vi "Preview.vi"(8 "error in (no error)":errorcluster, 10 "Project":refnum<vi>, 11 "IB_Tree_Item_Proj_Container in":refnum<class "IB_Tree_Item_Proj_Container.lvclass">) -> (0 "error out":errorcluster, 2 "first preview?":bool, 3 "IB_Tree_Item_Proj_Container out":refnum<class "IB_Tree_Item_Proj_Container.lvclass">)   [LabVIEW 2020, in "IB_Tree_Item_Proj_Container.lvclass"]
uses:
  <vilib>/AppBuilder/IB_Classes/Tree_Item_Proj_Container/IB_Tree_Item_Proj_Container.lvclass
  <vilib>/AppBuilder/IB_Classes/Tree_Item_Proj_Container/IB_Tree_Item_Proj_Container.lvclass/IB_Tree_Item_Proj_Container.ctl
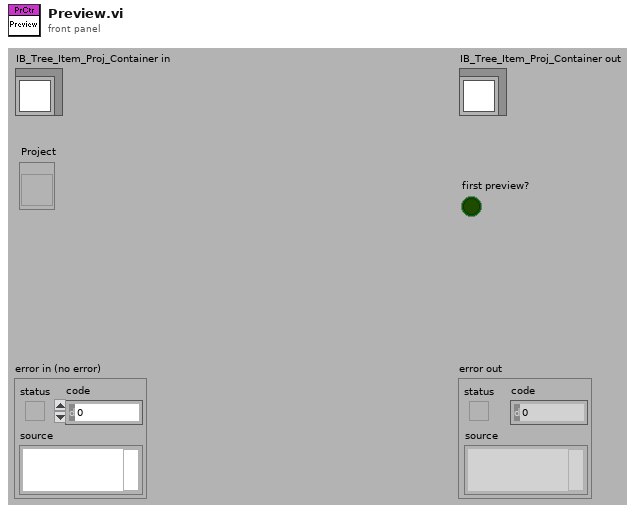
[diagram p1: front panel]
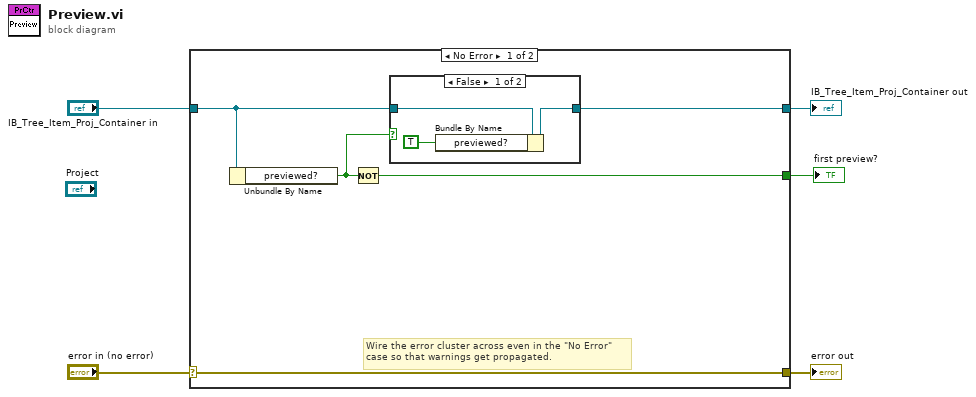
[diagram p0: block diagram]
diagram:
  n1 = case shown="No Error" "error in (no error)" {
    selector: "error in (no error)" -> [w10 w16]
    tunnel: [w10 w16] -> w4
    tunnel: [w8 w15] -> w2
    tunnel: "IB_Tree_Item_Proj_Container in" -> [w9 w15]
    tunnel: [w7 _] -> w1
    frame No Error {
      # "Wire the error cluster across even in the \"No Error\"\ncase so that warnings get propagated."
      n2 = Unbundle By Name(w9) -> ("previewed?"=w6:bool)
      n3 = Not(x=w6) -> (.not. x?=w7:bool)
      n4 = case shown="False" w6 {
        tunnel: w9 -> [w13 w14]
        tunnel: [w12 w14] -> w8
        frame False {
          n5 = Bundle By Name(cluster=w13, "previewed?"=TRUE ("data.previewed?")) -> (w12:refnum<class "IB_Tree_Item_Proj_Container.lvclass">)
        }
        frame True {
        }
      }
    }
    frame Error {
    }
  }
  "error out" <- w4
  "IB_Tree_Item_Proj_Container out" <- w2
  "first preview?" <- w1
